vi "FixNumber.vi"(5 "Decimals":u8, 9 "String in":string) -> (1 "value":dbl, 3 "String out":string)   [LabVIEW 2016]
doc: "This vi 'fixes' a numeric string.\nRemoves leading zeros, ensures there is a digit in front of a decimal place and after a - sign and limits number of decimal places.\nReturns the 'fixed' string and its numeric value.\n\nR.Gibson 13-Aug-2007"
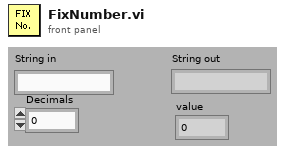
[diagram p1: front panel]
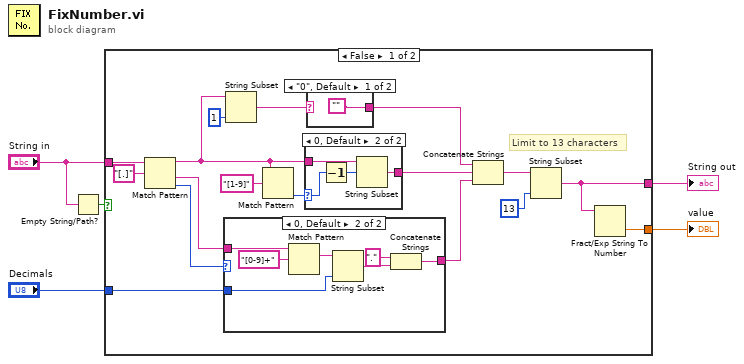
[diagram p0: block diagram]
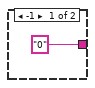
[diagram p3: hidden frame]
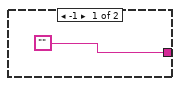
[diagram p4: hidden frame]
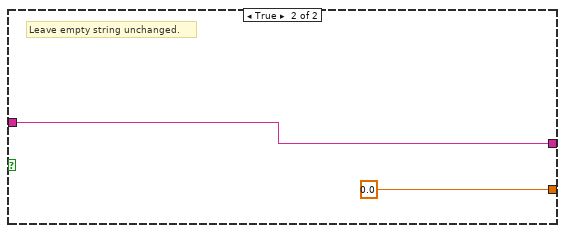
[diagram p5: hidden frame]
diagram:
  n1 = Empty String/Path?(string/path="String in") -> (empty?=w1:bool)
  n2 = case shown="False" w1 {
    tunnel: "String in" -> [w22 w39]
    tunnel: "Decimals" -> [w10 _]
    tunnel: [w9 0.0] -> w4
    tunnel: [w7 w39] -> w3
    frame False {
      # "Limit to 13 characters"
      n3 = Match Pattern(string=w22, regular expression="[.]") -> (before substring=w13:string, after substring=w20:string, offset past match=w19:i32)  [unwired: 2 out]
      n4 = case shown="0, Default" w19 {
        tunnel: w20 -> [_ w37]
        tunnel: ["" w35] -> w14
        tunnel: w10 -> [_ w31]
        frame -1 {
        }
        frame 0, Default {
          n5 = Match Pattern(string=w37, regular expression="[0-9]+") -> (match substring=w33:string)  [unwired: 4 out]
          n6 = String Subset(string=w33, length (rest)=w31) -> (substring=w32:string)  [unwired: 1 out]
          n7 = Concatenate Strings("." ("string"), w32) -> (w35:string)
        }
      }
      n8 = String Subset(string=w13, length (rest)=1 ("length (rest)")) -> (substring=w12:string)  [unwired: 1 out]
      n9 = Match Pattern(string=w13, regular expression="[1-9]") -> (offset past match=w15:i32)  [unwired: 4 out]
      n10 = case shown="0, Default" w15 {
        selector: w15 -> [_ w26]
        tunnel: w13 -> [_ w29]
        tunnel: ["0" ("String in") w28] -> w16
        frame -1 {
        }
        frame 0, Default {
          n11 = Decrement(x=w26) -> (x-1=w27:i32)
          n12 = String Subset(string=w29, offset (0)=w27) -> (substring=w28:string)  [unwired: 1 out]
        }
      }
      n13 = case shown="\"0\", Default" w12 {
        selector: w12 -> [_ w24]
        tunnel: ["" w24] -> w11
        frame "0", Default {
        }
        frame "-" {
        }
      }
      n14 = Concatenate Strings(w11, w16, w14) -> (w8:string)
      n15 = String Subset(string=w8, length (rest)=13 ("y")) -> (substring=w7:string)  [unwired: 1 out]
      n16 = Fract/Exp String To Number(string=w7) -> (number=w9:dbl)  [unwired: 4 out]
    }
    frame True {
      # "Leave empty string unchanged."
    }
  }
  "String out" <- w3
  "value" <- w4
